vi "OutbitsClearMemory.vi"   [LabVIEW 2014]
uses:
  <vilib>/rvi/Emulation/niFpgaGetClockAttributes.vi
  <vilib>/rvi/Emulation/niFpgaSctlEmulationGetInTimedLoop.vi
  <vilib>/rvi/Emulation/niFpgaEmulationReportErrorSimple.vi
  OutbitsGlobalVars.vi
  <vilib>/rvi/Memory/Memory_Emulation/nirvimemoryFastEmulation.vi
  <vilib>/rvi/Memory/Memory_Emulation/nirvimemoryEmulation.vi
  <vilib>/rvi/Emulation/niFpgaEmulationIsFPGAContextNoSignature.vi
  <vilib>/rvi/DataTransferAndStorage/Container/Common/niFpgaContainerGetUniqueNameForEmu.vi
  <vilib>/rvi/Emulation/niFpgaProcessEmulError.vi
  <vilib>/rvi/errors/nirviReportUnexpectedCaseInternalError (U32).vi
  <vilib>/rvi/Emulation/niFpgaCriticalErrorInLSC.vi
  <vilib>/rvi/DataTransferAndStorage/Container/XNode/niFpgaContainer.xnode
panel:
  # "This will write zeros to all memory addresses"
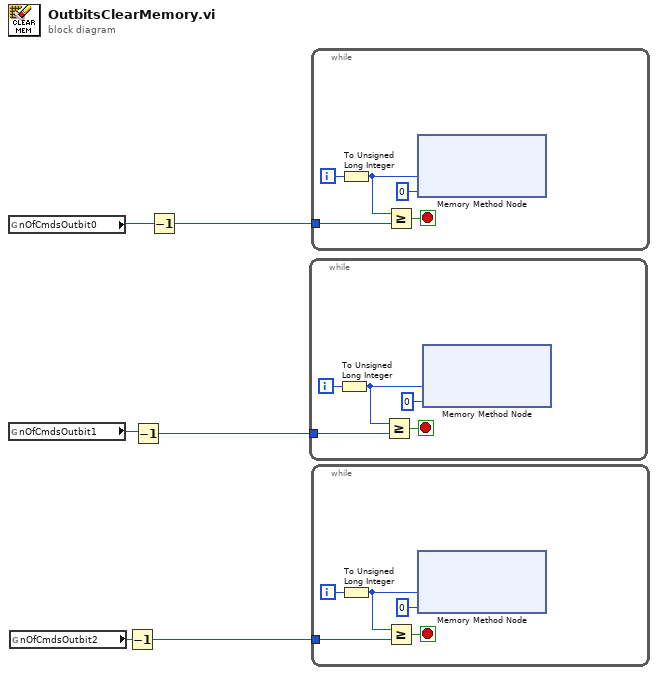
[diagram p0: block diagram]
diagram:
  n1 = global read "OutbitsGlobalVars.vi" "nOfCmdsOutbit0"() -> (w6:u32)
  n2 = global read "OutbitsGlobalVars.vi" "nOfCmdsOutbit1"() -> (w4:u32)
  n3 = global read "OutbitsGlobalVars.vi" "nOfCmdsOutbit2"() -> (w2:u32)
  n4 = Decrement(x=w2) -> (x-1=w1:u32)
  n5 = Decrement(x=w4) -> (x-1=w3:u32)
  n6 = Decrement(x=w6) -> (x-1=w5:u32)
  n7 = while {
    tunnel: w3 -> [w10]
    i -> [w11]
    stop <- w9 stop-if-true
    n8 = To Unsigned Long Integer(number=w11) -> (unsigned 32bit integer=w8:u32)
    n9 = Greater Or Equal?(x=w8, y=w10) -> (x >= y?=w9:bool)
    n10 = xnode ("Memory Method Node")("Address"=w8, "Data"=u32 0) -> ()  [unwired: 1 in, 1 out]
  }
  n11 = while {
    tunnel: w5 -> [w14]
    i -> [w16]
    stop <- w13 stop-if-true
    n12 = To Unsigned Long Integer(number=w16) -> (unsigned 32bit integer=w15:u32)
    n13 = Greater Or Equal?(x=w15, y=w14) -> (x >= y?=w13:bool)
    n14 = xnode ("Memory Method Node")("Address"=w15, "Data"=u32 0) -> ()  [unwired: 1 in, 1 out]
  }
  n15 = while {
    tunnel: w1 -> [w20]
    i -> [w21]
    stop <- w19 stop-if-true
    n16 = To Unsigned Long Integer(number=w21) -> (unsigned 32bit integer=w18:u32)
    n17 = Greater Or Equal?(x=w18, y=w20) -> (x >= y?=w19:bool)
    n18 = xnode ("Memory Method Node")("Address"=w18, "Data"=u32 0) -> ()  [unwired: 1 in, 1 out]
  }
